vi "POST.vi"(7 "LabVIEW Web Service Request":refnum<class "Web Request.lvclass">) -> ()   [LabVIEW 2015]
uses:
  <vilib>/wsapi/Web Request.lvclass
panel:
  out "sendToVI":string
  out "session ID cookie":string
  # "Use the Web Service Request input terminal to call the VIs on the Web Services palette. Do not remove it from the connector pane unless you don't need access to the palette."
  # "Each additional control wired to the connector pane will be available as an input in the URL. To include an indicator in terminal-mode output (the default setting), it must also be wired to the connector pane."
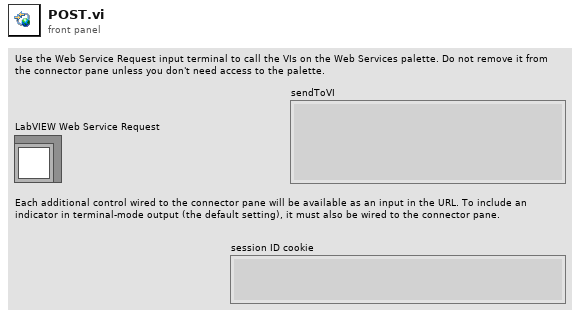
[diagram p1: front panel]
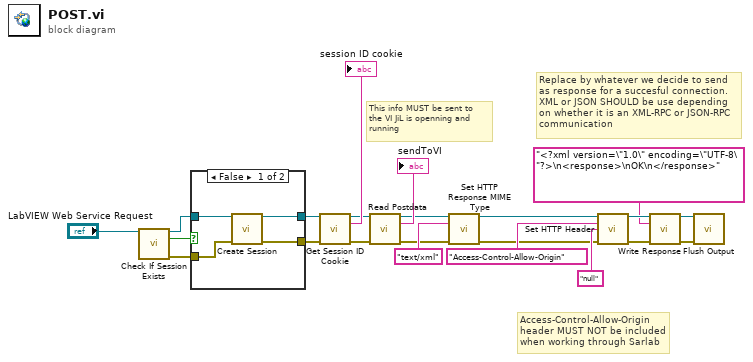
[diagram p0: block diagram]
diagram:
  # "This info MUST be sent to\nthe VI JiL is openning and\nrunning"
  # "Replace by whatever we decide to send\nas response for a succesful connection.\nXML or JSON SHOULD be use depending\non whether it is an XML-RPC or JSON-RPC\ncommunication"
  # "Access-Control-Allow-Origin\nheader MUST NOT be included when working through Sarlab"
  n1 = call <vilib>:"Check If Session Exists.vi"("LabVIEW Web Service Request"="LabVIEW Web Service Request") -> ("LabVIEW Web Service Request out"=w22:refnum<class "Web Request.lvclass">, "session exists?"=w21:bool, "error out"=w19:errorcluster)  [unwired: 12 in]
  n2 = case shown="False" w21 {
    tunnel: w22 -> [w26 w28]
    tunnel: [w25 w28] -> w20
    tunnel: w19 -> [w24 w27]
    tunnel: [w23 w27] -> w18
    frame False {
      n3 = call <vilib>:"Create Session.vi"("LabVIEW Web Service Request"=w26, "error in (no error)"=w24) -> ("LabVIEW Web Service Request out"=w25:refnum<class "Web Request.lvclass">, "error out"=w23:errorcluster)  [unwired: 11 in, 1 out]
    }
    frame True {
    }
  }
  n4 = call <vilib>:"Get Session ID Cookie.vi"("LabVIEW Web Service Request"=w20, "error in (no error)"=w18) -> ("LabVIEW Web Service Request out"=w15:refnum<class "Web Request.lvclass">, "session ID cookie"=→"session ID cookie":string, "error out"=w14:errorcluster)  [unwired: 11 in]
  n5 = call <vilib>:"Read Postdata.vi"("LabVIEW Web Service Request"=w15, "error in (no error)"=w14) -> ("LabVIEW Web Service Request out"=w4:refnum<class "Web Request.lvclass">, "postdata"=→"sendToVI":string, "error out"=w3:errorcluster)  [unwired: 11 in]
  n6 = call <vilib>:"Set HTTP Response MIME Type.vi"("LabVIEW Web Service Request"=w4, "MIME type (text/html)"="text/xml" ("header"), "error in (no error)"=w3) -> ("LabVIEW Web Service Request out"=w2:refnum<class "Web Request.lvclass">, "error out"=w1:errorcluster)  [unwired: 11 in]
  n7 = call <vilib>:"Set HTTP Header.vi"("LabVIEW Web Service Request"=w2, "header"="Access-Control-Allow-Origin", "header value"="null", "error in (no error)"=w1) -> ("LabVIEW Web Service Request out"=w10:refnum<class "Web Request.lvclass">, "error out"=w9:errorcluster)  [unwired: 10 in]
  n8 = call <vilib>:"Write Response.vi"("LabVIEW Web Service Request"=w10, "response string"="<?xml version=\"1.0\" encoding=\"UTF-8\"?>\n<response>\nOK\n</response>", "error in (no error)"=w9) -> ("LabVIEW Web Service Request out"=w7:refnum<class "Web Request.lvclass">, "error out"=w6:errorcluster)  [unwired: 11 in]
  n9 = call <vilib>:"Flush Output.vi"("LabVIEW Web Service Request"=w7, "error in (no error)"=w6) -> ()  [unwired: 12 in, 2 out]
